vi "GettingStarted_Gen_148X_FPGA.vi"() -> ()   [LabVIEW 2020, in "GettingStarted_Gen_148X_FPGA.lvlib"]
uses:
  GettingStarted_Gen_148X_FPGA.lvlib
  <vilib>/Platform/TimedLoop/XDataNode/wakeup.ctl
  <vilib>/Platform/TimedLoop/XDataNode/XDNodeRunTimeDep.lvlib
  <vilib>/Platform/TimedLoop/XDataNode/nitl_modes.ctl
  <vilib>/Platform/TimedLoop/XDataNode/timing_clust.ctl
  <vilib>/Platform/TimedLoop/XDataNode/XDataNode.xnode
  <vilib>/eio/EIONode/EIONode.xnode
  <instrlib>/FlexRIO/API/FPGA/v1/FlexRIO API FPGA v1.lvlib
  Common/GettingStarted_Common_148X_FPGA.lvlib
  <vilib>/rvi/eio/common/nirviEmuTemplateMethod_errors.vi
  <instrlib>/FlexRIO/CSI-2/v2/FPGA/NI CSI-2 API FPGA v2.lvlib
  <instrlib>/FlexRIO/CSI-2/v2/FPGA/DRAM Manager/Public/Partition Range.ctl
  <instrlib>/FlexRIO/CSI-2/v2/FPGA/DRAM Manager/DRAM Manager v2.lvlib
  Common/Types/DRAM Status.ctl
  Types/Serial Output Channel Status.ctl
  Types/Serial Output Channel Datapath Configuration.ctl
  <instrlib>/FlexRIO/CSI-2/v2/FPGA/Types/GPIO Bank.ctl
  Common/Types/SerDes Identifier.ctl
  <instrlib>/FlexRIO/CSI-2/v2/FPGA/Types/Generation Engine State.ctl
  Common/Types/Display Channel Status.ctl
  <instrlib>/FlexRIO/CSI-2/v2/Common/Types/LLP Data Type.ctl
  <instrlib>/FlexRIO/CSI-2/v2/Common/NI CSI-2 API Common v2.lvlib
  <instrlib>/FlexRIO/CSI-2/v2/FPGA/Types/Display Parameters.ctl
  Common/Types/GPIO User Bank.ctl
panel:
  in  "reset timestamp (strobe)":bool
  out "user gpio bank destination":T1
  in  "user gpio bank source":T1
  in  "gpio routes":i8[](array[numeric])=[-1, -1, -1, -1, -1, -1, -1, -1, -1, -1, -1, -1, -1, -1, -1, -1, -1, -1, -1, -1, -1, -1, -1, -1, -1, -1, -1, -1, -1, -1, -1, -1, -1, -1, -1, -1, -1, -1, -1, -1, -1, -1, -1, -1, -1, -1, -1, -1, -1, -1, -1, -1, -1, -1, -1, -1, -1, -1, -1, -1, -1, -1, -1, -1, -1, -1, -1, -1, -1, -1, -1, -1, -1, -1, -1, -1, -1, -1, -1, -1, -1, -1, -1, -1, -1, -1, -1, -1, -1, -1, -1, -1, -1, -1, -1, -1]
  out "user timestamp fifo overflow":bool
  out "gpio timestamp fifo overflow":bool
  out "serdes gpio bank input select valid":bool
  out "gpio bank input":T2
  in  "gpio bank input select":T3
  out "serdes gpio bank output select valid":bool
  in  "gpio bank output enable":T2
  in  "gpio bank output select":T3
  in  "gpio bank output":T2
  in  "serial channel display parameters":T4[](array[typedef])=[{"virtual channel"=0.0, "payload data type"=enum."Frame Start", "frame skip count"=0, "line skip count"=0, "pixel skip count"=0.0}, {"virtual channel"=0.0, "payload data type"=enum."Frame Start", "frame skip count"=0, "line skip count"=0, "pixel skip count"=0.0}, {"virtual channel"=0.0, "payload data type"=enum."Frame Start", "frame skip count"=0, "line skip count"=0, "pixel skip count"=0.0}, {"virtual channel"=0.0, "payload data type"=enum."Frame Start", "frame skip count"=0, "line skip count"=0, "pixel skip count"=0.0}, {"virtual channel"=0.0, "payload data type"=enum."Frame Start", "frame skip count"=0, "line skip count"=0, "pixel skip count"=0.0}, {"virtual channel"=0.0, "payload data type"=enum."Frame Start", "frame skip count"=0, "line skip count"=0, "pixel skip count"=0.0}, {"virtual channel"=0.0, "payload data type"=enum."Frame Start", "frame skip count"=0, "line skip count"=0, "pixel skip count"=0.0}, {"virtual channel"=0.0, "payload data type"=enum."Frame Start", "frame skip count"=0, "line skip count"=0, "pixel skip count"=0.0}]
  in  "display serial channel selectors":fxp<+,3,3>[](array[numeric])=[0.0, 0.0, 0.0, 0.0, 0.0, 0.0, 0.0, 0.0]
  in  "enabled display channels":bool[](array[boolean])=[FALSE, FALSE, FALSE, FALSE, FALSE, FALSE, FALSE, FALSE]
  out "display channel status":T6[](array[typedef])
  out "generation state":T7
  in  "channel configs":T8[](array[typedef])
  in  "sw start trigger":bool
  in  "stop trigger (strobe)":bool
  in  "enable sync pulse":bool
  in  "generate sync pulse (strobe)":bool
  out "channel status":T9[](array[typedef])
  out "flexrio.module.dram ready 0":bool
  out "flexrio.module.io ready 0":bool
  out "flexrio.module.io error 0":i32
  in  "dram partition configs":T11[](array[typedef])=[{"first address"=0, "last address"=0}, {"first address"=0, "last address"=0}, {"first address"=0, "last address"=0}, {"first address"=0, "last address"=0}, {"first address"=0, "last address"=0}, {"first address"=0, "last address"=0}, {"first address"=0, "last address"=0}, {"first address"=0, "last address"=0}]
  out "dram manager 1.num active streams":fxp<+,3,3>
  out "dram manager 0.num active streams":fxp<+,3,3>
  in  "dram arbiter config":T12={"write grant time (clocks)"=256, "read grant time (clocks)"=256}
  in  "write time slice":u16=256
  in  "request time slice":u16=256
  in  "reset (strobe)":bool
  # "Channel Configuration"
  # "GPIO Routing"
  # "User Timestamps"
  # "GPIO Control"
  # "Display Configuration"
  # "Trigger Control"
  # "Module Status"
  # "DRAM Manager Configuration"
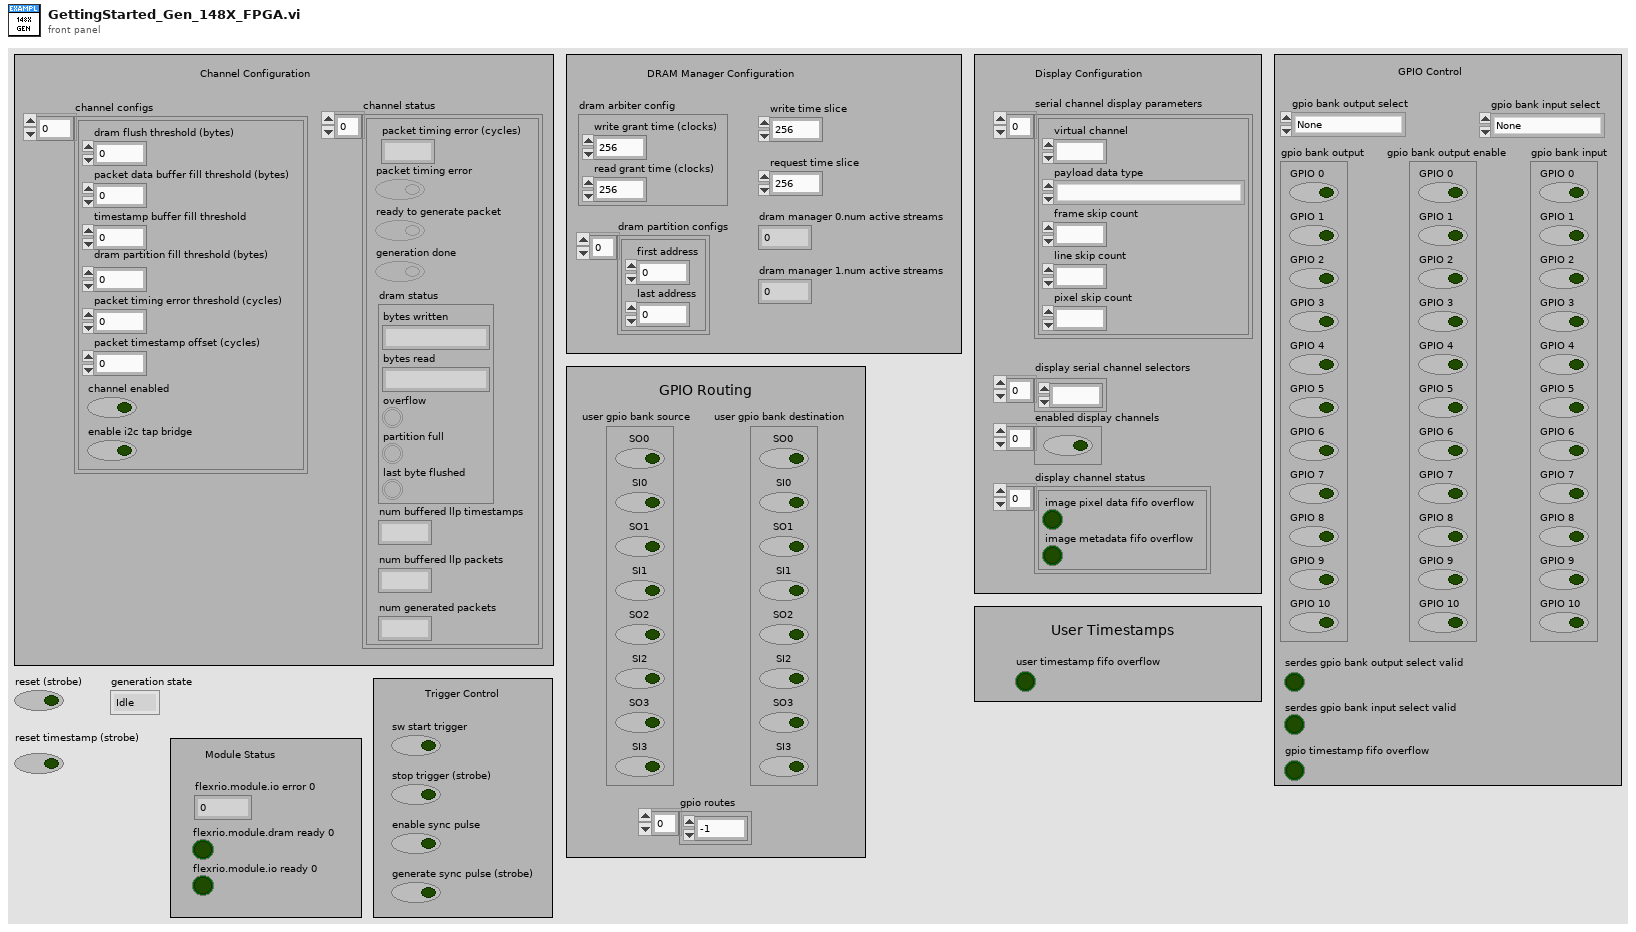
[diagram p1: front panel]
types:
  T1 = typedef "GettingStarted_Common_148X_FPGA.lvlib/GPIO User Bank.ctl" = cluster{"SO0":bool, "SI0":bool, "SO1":bool, "SI1":bool, "SO2":bool, "SI2":bool, "SO3":bool, "SI3":bool}
  T2 = typedef "NI CSI-2 API FPGA v2.lvlib/GPIO Bank.ctl" = cluster{"GPIO 0":bool, "GPIO 1":bool, "GPIO 2":bool, "GPIO 3":bool, "GPIO 4":bool, "GPIO 5":bool, "GPIO 6":bool, "GPIO 7":bool, "GPIO 8":bool, "GPIO 9":bool, "GPIO 10":bool}
  T3 = typedef "GettingStarted_Common_148X_FPGA.lvlib/SerDes Identifier.ctl" = enum8{"None", "SI 0 Deserializer", "SI 1 Deserializer", "SI 2 Deserializer", "SI 3 Deserializer", "SI 4 Deserializer", "SI 5 Deserializer", "SI 6 Deserializer", "SI 7 Deserializer", "SO 0 Serializer", "SO 1 Serializer", "SO 2 Serializer", "SO 3 Serializer", "SO 4 Serializer", "SO 5 Serializer", "SO 6 Serializer", "SO 7 Serializer", "SI 0 SI 1 Deserializer", "SI 2 SI 3 Deserializer", "SI 4 SI 5 Deserializer", "SI 6 SI 7 Deserializer"}
  T4 = typedef "NI CSI-2 API FPGA v2.lvlib/Display Parameters.ctl" = cluster{"virtual channel":fxp<+,4,4>, "payload data type":T5, "frame skip count":u16, "line skip count":u8, "pixel skip count":fxp<+,5,5>}
  T5 = typedef "NI CSI-2 API Common v2.lvlib/LLP Data Type.ctl" = enum8{"Frame Start", "Frame End", "Line Start", "Line End", "End of Transmission", "Reserved 0", "Reserved 1", "Reserved 2", "Generic Short Packet 1", "Generic Short Packet 2", "Generic Short Packet 3", "Generic Short Packet 4", "Generic Short Packet 5", "Generic Short Packet 6", "Generic Short Packet 7", "Generic Short Packet 8", "Null", "Blanking Data", "Embedded 8-bit non Image Data", "Generic Long Packet 1", "Generic Long Packet 2", "Generic Long Packet 3", "Generic Long Packet 4", "Reserved 3", "YUV420 8-bit", "YUV420 10-bit", "Legacy YUV420 8-bit", "Reserved 4", "YUV420 8-bit Chroma Shifted", "YUV420 10-bit Chroma Shifted", "YUV422 8-bit", "YUV422 10-bit", "RGB444", "RGB555", "RGB565", "RGB666", "RGB888", "Reserved 5", "Reserved 6", "RAW 24", "RAW 6", "RAW 7", "RAW 8", "RAW 10", "RAW 12", "RAW 14", "RAW 16", "RAW 20", "User Defined 8-bit Data 1", "User Defined 8-bit Data 2", "User Defined 8-bit Data 3", "User Defined 8-bit Data 4", "User Defined 8-bit Data 5", "User Defined 8-bit Data 6", "User Defined 8-bit Data 7", "User Defined 8-bit Data 8", "USL Command", "Reserved 7", "Reserved 8", "Reserved 9", "Reserved 10", "Reserved 11", "Reserved 12", "LRTE EPD Spacer"}
  T6 = typedef "GettingStarted_Common_148X_FPGA.lvlib/Display Channel Status.ctl" = cluster{"image pixel data fifo overflow":bool, "image metadata fifo overflow":bool}
  T7 = typedef "NI CSI-2 API FPGA v2.lvlib/Generation Engine State.ctl" = enum8{"Idle", "Ready For Start Trigger", "Generate Packets", "Done", "Error"}
  T8 = typedef "GettingStarted_Gen_148X_FPGA.lvlib/Serial Output Channel Datapath Configuration.ctl" = cluster{"dram flush threshold (bytes)":u64, "packet data buffer fill threshold (bytes)":u64, "timestamp buffer fill threshold":u32, "packet timing error threshold (cycles)":u64, "channel enabled":bool, "dram partition fill threshold (bytes)":u64, "enable i2c tap bridge":bool, "packet timestamp offset (cycles)":i64}
  T9 = typedef "GettingStarted_Gen_148X_FPGA.lvlib/Serial Output Channel Status.ctl" = cluster{"num buffered llp packets":fxp<+,14,14>, "packet timing error (cycles)":u64, "packet timing error":bool, "ready to generate packet":bool, "dram status":T10, "num buffered llp timestamps":u32, "generation done":bool, "num generated packets":u64}
  T10 = typedef "GettingStarted_Common_148X_FPGA.lvlib/DRAM Status.ctl" = cluster{"bytes written":u64, "bytes read":u64, "overflow":bool, "partition full":bool, "last byte flushed":bool}
  T11 = typedef "DRAM Manager v2.lvlib/Partition Range.ctl" = cluster{"first address":u32, "last address":u32}
  T12 = cluster{"write grant time (clocks)":u16, "read grant time (clocks)":u16}
  T13 = typedef "GettingStarted_Common_148X_FPGA.lvlib/Common Resources.ctl" = cluster{"sync pulse resources":T14, "serial channel resources":T15, "dram manager 0":T17, "dram manager 1":T17}
  T14 = typedef "NI CSI-2 API FPGA v2.lvlib/Sync Pulse Resources.ctl" = cluster{"sync pulse destination terminal":refnum<k21>, "sync100":refnum<k21>, "sync pulse source terminal":refnum<k21>, "imported sync pulse register":refnum<k21>, "generate sync pulse handshake":refnum<k21>, "enable sync pulse register":refnum<k21>, "sync pulse clock":refnum<k21>}
  T15 = typedef "GettingStarted_Common_148X_FPGA.lvlib/Serial Channel Resources.ctl" = cluster{"sc 0":T16, "sc 1":T16, "sc 2":T16, "sc 3":T16, "sc 4":T16, "sc 5":T16, "sc 6":T16, "sc 7":T16}
  T16 = typedef "GettingStarted_Common_148X_FPGA.lvlib/Single Serial Channel Resources.ctl" = cluster{"completed frames register":refnum<k21>}
  T17 = typedef "DRAM Manager v2.lvlib/DRAM Manager.ctl" = cluster{"DRAM class":refnum<class "niInstr Memory DRAM v1 FPGA.lvclass">, "process clock":refnum<k21>, "registers":T18, "FIFOs":T20, "num active streams":fxp<+,3,3>, "max open read requests":u16}
  T18 = typedef "DRAM Manager v2.lvlib/DRAM Manager Registers.ctl" = cluster{"configuration":cluster{"write time slice":refnum<k21>, "request time slice":refnum<k21>, "DRAM arbiter config":refnum<k21>, "partition config":refnum<k21>}, "reset":cluster{"handshake":T19, "process":cluster{"in":refnum<k21>, "out":refnum<k21>}, "write":cluster{"in":refnum<k21>, "out 0":refnum<k21>, "out 1":refnum<k21>, "out 2":refnum<k21>, "out 3":refnum<k21>}, "read":cluster{"in":refnum<k21>, "out 0":refnum<k21>, "out 1":refnum<k21>, "out 2":refnum<k21>, "out 3":refnum<k21>}}, "status":cluster{"partition full":refnum<k21>}}
  T19 = typedef "DRAM Manager v2.lvlib/Handshake Registers.ctl" = cluster{"start.go":refnum<k21>, "start.go rcvd":refnum<k21>, "done.go":refnum<k21>, "done.go rcvd":refnum<k21>}
  T20 = typedef "DRAM Manager v2.lvlib/DRAM Manager FIFOs.ctl" = cluster{"write data":cluster{"FIFO 0":T21, "FIFO 1":T21, "FIFO 2":T21, "FIFO 3":T21}, "request metadata":cluster{"FIFO":T22}, "read data VOQ":cluster{"FIFO 0":T23, "FIFO 1":T23, "FIFO 2":T23, "FIFO 3":T23}, "read data":cluster{"FIFO 0":T23, "FIFO 1":T23, "FIFO 2":T23, "FIFO 3":T23}}
  T21 = typedef "DRAM Manager v2.lvlib/Write Data FIFO Ref.ctl" = refnum<k21>
  T22 = typedef "DRAM Manager v2.lvlib/Read Request Metadata FIFO Ref.ctl" = refnum<k21>
  T23 = typedef "DRAM Manager v2.lvlib/Read Data FIFO Ref.ctl" = refnum<k21>
  T24 = typedef "XDNodeRunTimeDep.lvlib/timing_clust.ctl" = cluster{"Expected End [f-1]":u64, "Actual End [f-1]":u64, "Finished Late? [f-1]":bool, "Expected End [i-1]":u64, "Actual End [i-1]":u64, "Finished Late? [i-1]":bool, "Expected Start [i]":u64, "Actual Start [i]":u64, "Expected Start [f]":u64, "Actual Start [f]":u64, "Source Name":string, "Structure Name":string, "Period":i64, "Deadline":i64, "Offset":i64, "Start":i64, "Priority":i32, "Timeout":i32, "Mode":T25, "Wakeup Reason":T26, "Error":errorcluster, "Source Type":string, "Secondary Source Type":string, "Global End Time":u64, "Global Start Time":u64, "Frame Duration":u64, "Iteration Duration":u64, "Assigned CPU":i32, "I/O Scan Engine Mode":u32}
  T25 = typedef "XDNodeRunTimeDep.lvlib/nitl_modes.ctl" = enum32{"No Change", "Process missed periods, maintain original phase", "Discard missed periods, maintain original phase", "Process missed periods, ignore original phase", "Discard missed periods, ignore original phase"}
  T26 = typedef "XDNodeRunTimeDep.lvlib/wakeup.ctl" = enum32{"Normal", "Aborted", "Asynchronous wakeup", "Timing source error", "Timed loop error", "Timeout"}
  T27 = typedef "GettingStarted_Common_148X_FPGA.lvlib/GPIO Bank Output Configuration.ctl" = cluster{"gpio bank":T2, "gpio bank output enable":T2}
  T28 = typedef "GettingStarted_Common_148X_FPGA.lvlib/Tagged LLP Packets Cluster.ctl" = cluster{"tagged llp packet 0":T29, "tagged llp packet 1":T29, "tagged llp packet 2":T29, "tagged llp packet 3":T29, "tagged llp packet 4":T29, "tagged llp packet 5":T29, "tagged llp packet 6":T29, "tagged llp packet 7":T29}
  T29 = typedef "NI CSI-2 API FPGA v2.lvlib/Tagged LLP Packet.ctl" = cluster{"tag":T30, "llp packet":T34}
  T30 = typedef "NI CSI-2 API FPGA v2.lvlib/FPGA LLP Packet Tag.ctl" = cluster{"timestamp":T31, "size":T33}
  T31 = typedef "NI CSI-2 API FPGA v2.lvlib/FPGA LLP Packet Timestamp.ctl" = cluster{"valid":bool, "count":fxp<+,50,50>, "id":T32, "metadata":u8}
  T32 = typedef "NI CSI-2 API FPGA v2.lvlib/Timestamp ID.ctl" = enum8{"SI0 LLP", "SI1 LLP", "SI2 LLP", "SI3 LLP", "SI4 LLP", "SI5 LLP", "SI6 LLP", "SI7 LLP", "SO0 LLP", "SO1 LLP", "SO2 LLP", "SO3 LLP", "SO4 LLP", "SO5 LLP", "SO6 LLP", "SO7 LLP", "Ser0 GPIO Bank", "Ser1 GPIO Bank", "Ser2 GPIO Bank", "Ser3 GPIO Bank", "Ser4 GPIO Bank", "Ser5 GPIO Bank", "Ser6 GPIO Bank", "Ser7 GPIO Bank", "Des0 GPIO Bank", "Des1 GPIO Bank", "Des2 GPIO Bank", "Des3 GPIO Bank", "Des4 GPIO Bank", "Des5 GPIO Bank", "Des6 GPIO Bank", "Des7 GPIO Bank", "User0", "User1", "User2", "User3", "User4", "User5", "User6", "User7", "User8", "User9", "User10", "User11", "User12", "User13", "User14", "User15", "User16", "User17", "User18", "User19", "User20", "User21", "User22", "User23", "User24", "User25", "User26", "User27", "User28", "User29", "User30", "User31"}
  T33 = typedef "NI CSI-2 API FPGA v2.lvlib/FPGA LLP Packet Size.ctl" = cluster{"bytes":fxp<+,17,17>, "valid":bool}
  T34 = typedef "NI CSI-2 API FPGA v2.lvlib/LLP Packet.ctl" = cluster{"header":T35, "header valid":bool, "payload":T36, "payload valid":bool, "footer":T37, "footer valid":bool, "end of packet":bool}
  T35 = typedef "NI CSI-2 API FPGA v2.lvlib/LLP Packet Header.ctl" = cluster{"word count":u16, "ecc":fxp<+,6,6>, "vcx":fxp<+,2,2>, "data type":fxp<+,6,6>, "vc":fxp<+,2,2>}
  T36 = typedef "NI CSI-2 API FPGA v2.lvlib/LLP Packet Payload.ctl" = cluster{"end of payload":bool, "end of payload index":fxp<+,3,3>, "payload data":u8[]}
  T37 = typedef "NI CSI-2 API FPGA v2.lvlib/LLP Packet Footer.ctl" = cluster{"crc":u16}
  T38 = typedef "NI CSI-2 API FPGA v2.lvlib/Timestamp Counter Value.ctl" = cluster{"counter value":u64, "valid":bool}
  T39 = typedef "FlexRIO 148x FPGA v1.lvlib/i2c monitor.ctl" = cluster{"monitor word":u8, "is header?":bool, "read/write_n":bool, "ack":bool, "start":bool, "stop":bool, "valid":bool}
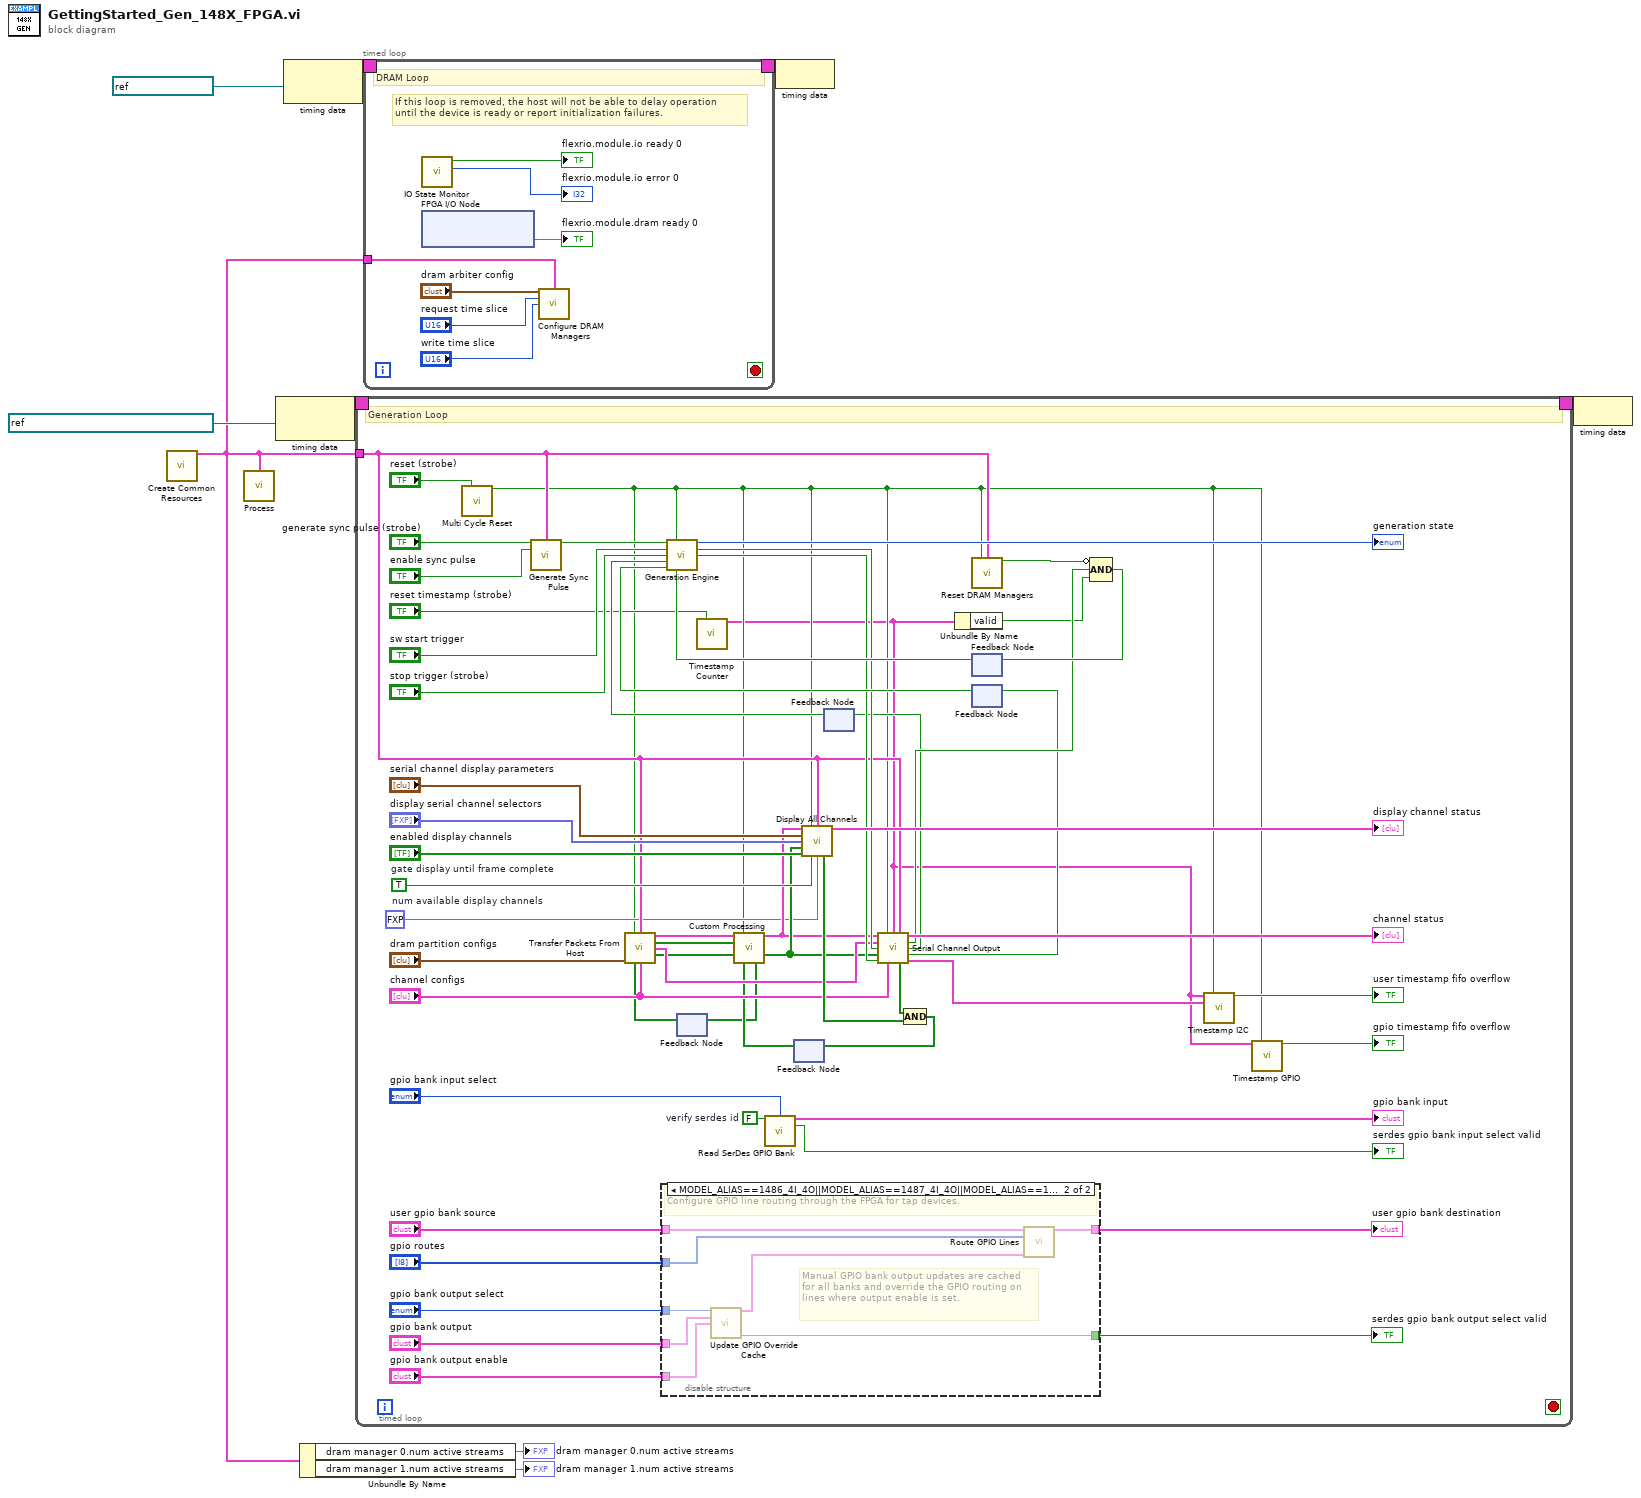
[diagram p0: block diagram]
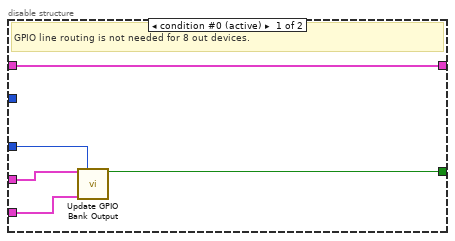
[diagram p2: hidden frame]
diagram:
  n1 = call "Create Common Resources.vi"() -> ("common resources"=w1:T13)  [unwired: 15 in]
  n2 = call "Process.vi"("resources"=w1) -> ()  [unwired: 15 in]
  n3 = node-c288(refnum<k21> "IO Socket\\CSI-2 AXI Stream Clock" ("Source Name")) -> (w6:T24)
  n4 = node-c288(refnum<k21> "80 MHz Clock" ("Source Name")) -> (w9:T24)
  n5 = Unbundle By Name(w1) -> ("dram manager 0.num active streams"=→"dram manager 0.num active streams":fxp<+,3,3>, "dram manager 1.num active streams"=→"dram manager 1.num active streams":fxp<+,3,3>)
  n6 = timed-loop {
    timing: w6 -> [_]
    timing-out: [_] -> w5
    tunnel: w1 -> [w33]
    stop <- _ stop-if-true
    w15 = fxp<+,4,4> 2.0  # num available display channels
    w40 = TRUE  # gate display until frame complete
    w49 = FALSE  # verify serdes id
    # "Generation Loop"
    n7 = call "Multi Cycle Reset.vi"("reset (strobe)"="reset (strobe)") -> ("reset (fanout)"=w13:bool)  [unwired: 14 in]
    n8 = call "Generate Sync Pulse.vi"("generate sync pulse (strobe)"="generate sync pulse (strobe)", "resources"=w33, "enable sync pulse"="enable sync pulse") -> ("sync pulse out"=w60:bool)  [unwired: 12 in]
    n9 = disable-structure shown="MODEL_ALIAS==1486_4I_4O||MODEL_ALIAS==1487_4I_4O||MODEL_ALIAS==1488_4I_4O||MODEL_ALIAS==1489_2I_2O" {
      disable-tunnel: "gpio bank output enable" -> [w71 w77]
      disable-tunnel: "gpio bank output" -> [w70 w78]
      disable-tunnel: "gpio bank output select" -> [w69 w79]
      disable-tunnel: [w68 w76] -> w27
      disable-tunnel: "gpio routes" -> [_ w74]
      disable-tunnel: "user gpio bank source" -> [w67 w73]
      disable-tunnel: [w67 w72] -> w24
      frame condition #0 (active) {
        # "GPIO line routing is not needed for 8 out devices."
        n10 = call "Update GPIO Bank Output.vi"("gpio bank"=w70, "gpio bank serdes id"=w69, "gpio bank output enable"=w71) -> ("serdes id valid"=w68:bool)  [unwired: 12 in]
      }
      frame condition #1 {
        # "Manual GPIO bank output updates are cached for all banks and override the GPIO routing on lines where output enable is set."
        # "Configure GPIO line routing through the FPGA for tap devices."
        n11 = call "Update GPIO Override Cache.vi"("override gpio bank serdes id"=w79, "override gpio bank"=w78, "override gpio bank output enable"=w77) -> ("gpio override cache"=w75:T27[], "valid override serdes id"=w76:bool)  [unwired: 11 in]
        n12 = call "Route GPIO Lines.vi"("user gpio bank in"=w73, "gpio routes"=w74, "override gpio bank ouptut configs"=w75) -> ("user gpio bank out"=w72:T1)  [unwired: 12 in]
      }
    }
    "serdes gpio bank output select valid" <- w27
    "user gpio bank destination" <- w24
    n13 = feedback #1() -> (w17:bool[])  [unwired: 1 in]
    n14 = call "Transfer Packets From Host.vi"("reset"=w13, "common resources"=w33, "dram partition configs"="dram partition configs", "ready for output"=w17, "channel configs"="channel configs") -> ("tagged llp packets cluster"=w23:T28, "end of data"=w16:bool[], "dram status"=w32:T10[], "output valid"=w22:bool[])  [unwired: 7 in]
    n15 = call <instrlib>:"Timestamp Counter.vi"("reset and start"="reset timestamp (strobe)") -> ("timestamp counter value"=w11:T38)  [unwired: 14 in]
    n16 = call "Read SerDes GPIO Bank.vi"("verify serdes id"=w49, "serdes id"="gpio bank input select") -> ("gpio bank input"=→"gpio bank input":T2, "serdes id valid"=→"serdes gpio bank input select valid":bool)  [unwired: 12 in]
    n17 = feedback #2() -> (w19:bool[])  [unwired: 1 in]
    n18 = call "Custom Processing.vi"("tagged llp packets cluster in"=w23, "reset"=w13, "end of data"=w16, "input valid"=w22, "ready for output"=w19) -> ("tagged llp packets cluster out"=w20:T28, "output valid"=w21:bool[], "ready for input"=w18:bool[])  [unwired: 7 in, 1 out]
    n19 = feedback-in #1(w18) -> ()
    n20 = call "Display All Channels.vi"("tagged llp packets cluster"=w20, "reset"=w13, "common resources"=w33, "serial channel display parameters"="serial channel display parameters", "display serial channel selectors"="display serial channel selectors", "input valid"=w21, "enabled display channels"="enabled display channels", "gate display until frame complete"=w40, "num available display channels"=w15) -> ("display channel status"=→"display channel status":T6[], "ready for input"=w43:bool[])  [unwired: 5 in]
    n21 = feedback #3() -> (w57:bool)  [unwired: 1 in]
    n22 = Unbundle By Name(w11) -> ("valid"=w10:bool)
    n23 = call "Reset DRAM Managers.vi"("reset"=w13, "resources"=w33) -> ("in reset"=w63:bool)  [unwired: 13 in]
    n24 = feedback #4() -> (w62:bool)  [unwired: 1 in]
    n25 = feedback #5() -> (w56:bool)  [unwired: 1 in]
    n26 = call "Generation Engine.vi"("synchronous start trigger"=w60, "reset"=w13, "sw start trigger"="sw start trigger", "stop trigger in"="stop trigger (strobe)", "packet timing error detected"=w57, "generation done"=w56, "ready for start trigger"=w62) -> ("generation state"=→"generation state":T7, "start"=w38:bool, "stop"=w39:bool)  [unwired: 6 in]
    n27 = call "Serial Channel Output.vi"("tagged llp packets cluster"=w20, "reset"=w13, "global counter"=w11, "common resources"=w33, "dram status"=w32, "start trigger"=w38, "output valid"=w21, "stop trigger"=w39, "channel configs"="channel configs") -> ("serial output channel status"=→"channel status":T9[], "ready for start trigger"=w37:bool, "packet timing error detected"=w35:bool, "generation done"=w34:bool, "ready for input"=w42:bool[], "i2c monitor array"=w36:T39[])  [unwired: 1 in]
    n28 = feedback-in #3(w35) -> ()
    n29 = Compound Arithmetic op=AND(w42, w43) -> (w41:bool[])
    n30 = feedback-in #2(w41) -> ()
    n31 = feedback-in #5(w34) -> ()
    n32 = Compound Arithmetic op=AND(invert w63, w37, w10) -> (w58:bool)
    n33 = feedback-in #4(w58) -> ()
    n34 = call "Timestamp I2C.vi"("timestamp counter value"=w11, "reset"=w13, "i2c monitor array"=w36) -> ("user timestamp fifo overflow"=→"user timestamp fifo overflow":bool)  [unwired: 12 in]
    n35 = call "Timestamp GPIO.vi"("timestamp counter value"=w11, "reset"=w13) -> ("gpio timestamp fifo overflow"=→"gpio timestamp fifo overflow":bool)  [unwired: 13 in]
  }
  n36 = timed-loop {
    timing: w9 -> [_]
    timing-out: [_] -> w8
    tunnel: w1 -> [w88]
    stop <- _ stop-if-true
    # "If this loop is removed, the host will not be able to delay operation \nuntil the device is ready or report initialization failures."
    # "DRAM Loop"
    n37 = call <instrlib>:"IO State Monitor.vi"() -> ("flexrio.module.io error 0"=→"flexrio.module.io error 0":i32, "flexrio.module.io ready 0"=→"flexrio.module.io ready 0":bool)  [unwired: 10 in]
    n38 = xnode "FPGA I/O Node"() -> ("DRAM Ready"=→"flexrio.module.dram ready 0")  [unwired: 1 in, 1 out]
    n39 = call "Configure DRAM Managers.vi"("dram arbiter config"="dram arbiter config", "resources"=w88, "request time slice"="request time slice", "write time slice"="write time slice") -> ()  [unwired: 12 in]
  }
  n40 = node-c288(w8) -> ()
  n41 = node-c288(w5) -> ()
